vi "SMTP Email Format Header Field.vi"(4 "character set":string, 5 "translit":string, 6 "header content":string="Der Müller und ein müdes Mädchen", 7 "header name (Subject: )":string="Subject: ") -> (0 "real charset":string, 3 "encoded header line":string)   [LabVIEW 2011, in "NewNI_SMTPEmail.lvlib"]
doc: "Formats an email header field to make it MIME and SMTP-compliant.\n\nIn particular, if escapes non-ASCII characters as quoted printables (RFC1522). The header content is truncated at the first EOLN character."
uses:
  NewNI_SMTPEmail.lvlib
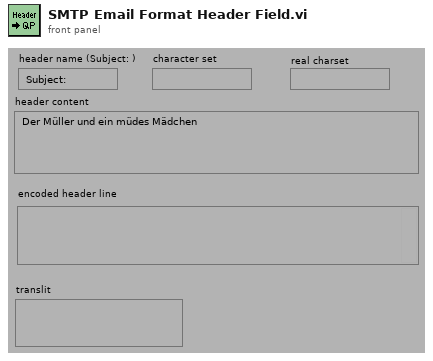
[diagram p1: front panel]
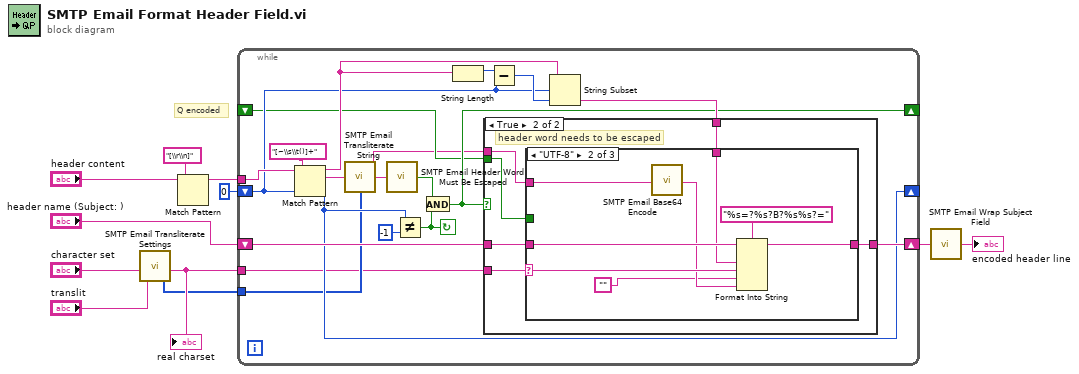
[diagram p0: block diagram]
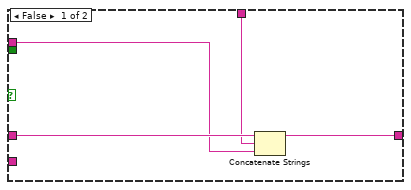
[diagram p2: hidden frame]
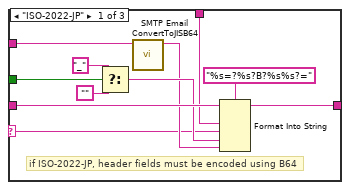
[diagram p3: hidden frame]
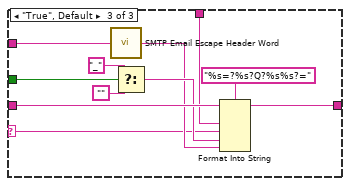
[diagram p4: hidden frame]
diagram:
  # "Q encoded"
  n1 = call "SMTP Email Transliterate Settings.vi"("transliteration"="translit", "character set"="character set") -> ("map"=w1:u8[], "charset out"=w2:string)  [unwired: 4 out]
  "real charset" <- w2
  n2 = Match Pattern(string="header content", regular expression="[\\r\\n]") -> (before substring=w10:string)  [unwired: 4 out]
  n3 = while {
    shift-left: _ -> [w16]
    shift-right: [w17] -> _
    tunnel: w1 -> [w18]
    tunnel: w2 -> [w13]
    tunnel: w10 -> [w27]
    shift-left: "header name (Subject: )" -> [w30]
    shift-right: [w21] -> w7
    shift-left: 0 -> [w19]
    shift-right: [w20] -> _
    stop <- w24 continue-if-true
    n4 = Match Pattern(string=w27, regular expression="[~\\s\\t()]+", offset (0)=w19) -> (before substring=w29:string, match substring=w26:string, offset past match=w20:i32)  [unwired: 1 out]
    n5 = call "SMTP Email Transliterate String.vi"("text in"=w26, "map"=w18) -> ("text out"=w12:string)
    n6 = call "SMTP Email Header Word Must Be Escaped.vi"("word"=w12) -> ("escape word"=w14:bool)
    n7 = Not Equal?(x=w20, y=-1) -> (x != y?=w24:bool)
    n8 = And(x=w14, y=w24) -> (x .and. y?=w17:bool)
    n9 = String Length(string=w29) -> (length=w28:i32)
    n10 = Subtract(x=w28, y=w19) -> (x-y=w23:i32)
    n11 = String Subset(string=w29, offset (0)=w19, length (rest)=w23) -> (substring=w22:string)
    n12 = case shown="True" w17 {
      tunnel: w30 -> [w34 w39]
      tunnel: w22 -> [w33 w37]
      tunnel: [w32 w38] -> w21
      tunnel: w13 -> [_ w35]
      tunnel: w16 -> [_ w40]
      tunnel: w12 -> [w31 w36]
      frame False {
        n13 = Concatenate Strings(w34, w33, w31) -> (w32:string)
      }
      frame True {
        # "header word needs to be escaped"
        n14 = case shown="\"UTF-8\"" w35 {
          selector: w35 -> [w41 w55 w60]
          tunnel: w40 -> [w42 _ w70]
          tunnel: w39 -> [w48 w58 w66]
          tunnel: [w47 w57 w65] -> w38
          tunnel: w37 -> [w46 w56 w64]
          tunnel: w36 -> [w44 w54 w62]
          frame "ISO-2022-JP" {
            # "if ISO-2022-JP, header fields must be encoded using B64"
            n15 = Select(t="_", s=w42, f="") -> (s? t:f=w45:string)
            n16 = call "SMTP Email ConvertToJISB64.vi"("data in"=w44) -> ("data out"=w43:string)  [unwired: 1 in, 9 out]
            n17 = Format Into String(format string="%s=?%s?B?%s%s?=", initial string=w48, w46, w41, w45, w43) -> (resulting string=w47:string)  [unwired: 1 in, 1 out]
          }
          frame "UTF-8" {
            n18 = call "SMTP Email Base64 Encode.vi"("Normal String"=w54) -> ("Base64 String"=w53:string)  [unwired: 1 in]
            n19 = Format Into String(format string="%s=?%s?B?%s%s?=", initial string=w58, w56, w55, "", w53) -> (resulting string=w57:string)  [unwired: 1 in, 1 out]
          }
          frame "True", Default {
            n20 = call "SMTP Email Escape Header Word.vi"("string"=w62) -> ("formated string"=w61:string)
            n21 = Select(t="_", s=w70, f="") -> (s? t:f=w63:string)
            n22 = Format Into String(format string="%s=?%s?Q?%s%s?=", initial string=w66, w64, w60, w63, w61) -> (resulting string=w65:string)  [unwired: 1 in, 1 out]
          }
        }
      }
    }
  }
  n23 = call "SMTP Email Wrap Subject Field.vi"("Subject in"=w7) -> ("Subject out"=→"encoded header line":string)
